vi "Archivos_TDMS.vi"() -> ()   [LabVIEW 2016]
panel:
  in  "file path":path
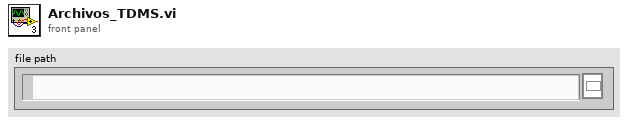
[diagram p1: front panel]
types:
  T1 = enum16{"open", "open or create", "create or replace", "create", "open (read-only)"}
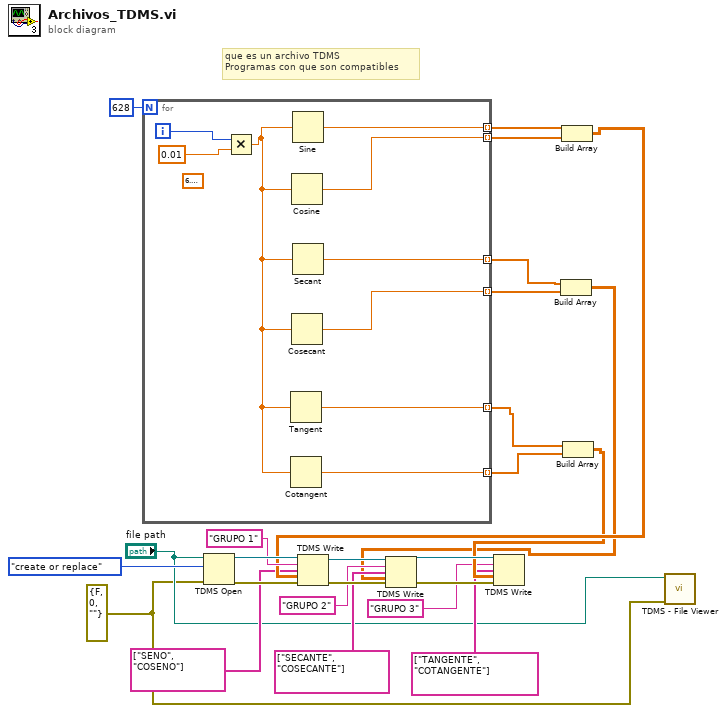
[diagram p0: block diagram]
diagram:
  w1 = errorcluster {"status"=FALSE, "code"=0, "source"=""} ("error in (no error)")
  # "que es un archivo TDMS\nProgramas con que son compatibles"
  n1 = for {
    N: 628 -> [_]
    tunnel: [w31] -> w24 mode=indexing
    tunnel: [w30] -> w23 mode=indexing
    tunnel: [w29] -> w22 mode=indexing
    tunnel: [w28] -> w21 mode=indexing
    tunnel: [w27] -> w20 mode=indexing
    tunnel: [w26] -> w19 mode=indexing
    i -> [w33]
    (unwired) 6.283185307179586
    n2 = Multiply(x=w33, y=0.01) -> (x*y=w32:dbl)
    n3 = Tangent(1:w32) -> (0:w27:dbl)
    n4 = Cotangent(1:w32) -> (0:w26:dbl)
    n5 = Cosine(x=w32) -> (cos(x)=w30:dbl)
    n6 = Cosecant(1:w32) -> (0:w28:dbl)
    n7 = Sine(x=w32) -> (sin(x)=w31:dbl)
    n8 = Secant(1:w32) -> (0:w29:dbl)
  }
  n9 = TDMS Open(8:w1, 10:T1."create or replace" ("operation (0:open)"), 11:"file path") -> (0:w16:errorcluster, 3:w17:refnum<k34>)  [unwired: 4 in]
  n10 = Build Array(w22, w21) -> (w5:dbl[][])
  n11 = Build Array(w24, w23) -> (w14:dbl[][])
  n12 = TDMS Write(0:w17, 5:"GRUPO 1" ("group name in (Untitled)"), 7:string[] ["SENO", "COSENO"] ("channel name(s) in (Untitled)"), 9:w14, 11:w16) -> (4:w12:refnum<k34>, 15:w11:errorcluster)  [unwired: 1 in, 2 out]
  n13 = TDMS Write(0:w12, 5:"GRUPO 2" ("group name in (Untitled)"), 7:string[] ["SECANTE", "COSECANTE"] ("channel name(s) in (Untitled)"), 9:w5, 11:w11) -> (4:w8:refnum<k34>, 15:w7:errorcluster)  [unwired: 1 in, 2 out]
  n14 = Build Array(w20, w19) -> (w6:dbl[][])
  n15 = TDMS Write(0:w8, 5:"GRUPO 3" ("group name in (Untitled)"), 7:string[] ["TANGENTE", "COTANGENTE"] ("channel name(s) in (Untitled)"), 9:w6, 11:w7) -> ()  [unwired: 1 in, 4 out]
  n16 = call <vilib>:"TDMS - File Viewer.vi"("error in (no error)"=w1, "file path"="file path") -> ()  [unwired: 4 in, 2 out]
